vi "DeviceReadStatus.vi"(8 "error in (no error)":errorcluster, 11 "DeviceLoopData in":T1) -> (0 "error out":errorcluster, 1 "Data":variant, 2 "Status":string, 3 "DeviceLoopData out":T1, 4 "Up To Date":bool, 6 "Ready":bool)   [LabVIEW 2015]
uses:
  <vilib>/ErrorRing/Error Ring.xnode
  <vilib>/Utility/error.llb/Error Cluster From Error Code.vi
  NetworkStream/NetworkStreamData.ctl
  DeviceLoopData.ctl
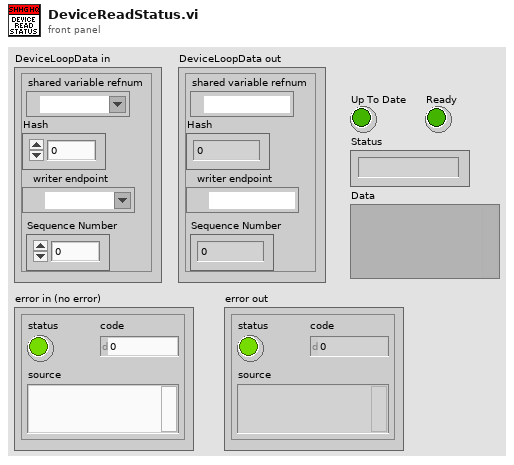
[diagram p1: front panel]
types:
  T1 = typedef "DeviceLoopData.ctl" = cluster{"shared variable refnum":refnum<k21>, "Hash":u64, "writer endpoint":refnum<k21>, "Sequence Number":u64}
  T2 = typedef "NetworkStream.lvlib/NetworkStreamData.ctl" = cluster{"Command/Status":string, "Data":variant, "Session Hash":u64, "Sequence Number":u64}
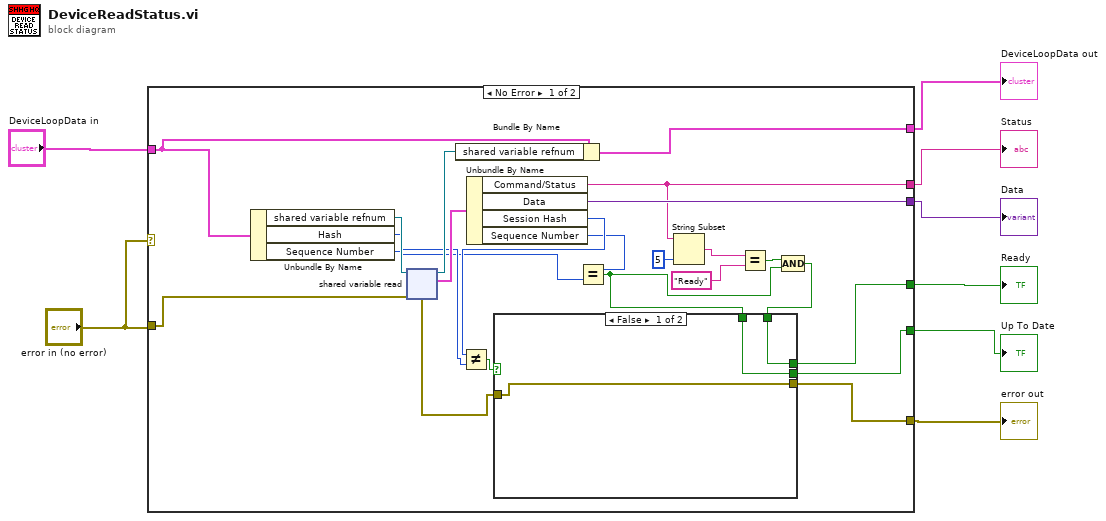
[diagram p0: block diagram]
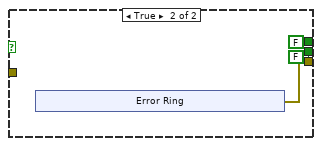
[diagram p2: hidden frame]
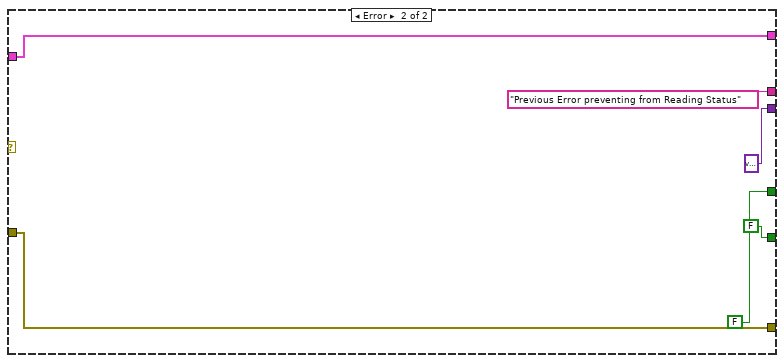
[diagram p3: hidden frame]
diagram:
  n1 = case shown="No Error" "error in (no error)" {
    tunnel: [w23 w48] -> w8
    tunnel: "error in (no error)" -> [w30 w48]
    tunnel: [w20 w46] -> w6
    tunnel: [w13 "Previous Error preventing from Reading Status" ("Command/Status")] -> w5
    tunnel: [w19 variant ("Data")] -> w4
    tunnel: [w10 FALSE] -> w3
    tunnel: "DeviceLoopData in" -> [w18 w46]
    tunnel: [w11 FALSE] -> w1
    frame No Error {
      n2 = Unbundle By Name(w18) -> ("shared variable refnum"=w28:refnum<k21>, "Hash"=w25:u64, "Sequence Number"=w21:u64)
      n3 = shared-variable-read(w28, w30) -> (w31:refnum<k21>, w24:errorcluster, w29:T2)
      n4 = Bundle By Name(cluster=w18, "shared variable refnum"=w31) -> (w20:T1)
      n5 = Unbundle By Name(w29) -> ("Command/Status"=w13:string, "Data"=w19:variant, "Session Hash"=w26:u64, "Sequence Number"=w22:u64)
      n6 = Not Equal?(x=w26, y=w25) -> (x != y?=w27:bool)
      n7 = Equal?(x=w22, y=w21) -> (x = y?=w9:bool)
      n8 = String Subset(string=w13, length (rest)=5 ("length (rest)")) -> (substring=w16:string)  [unwired: 1 in]
      n9 = Equal?(x=w16, y="Ready") -> (x = y?=w14:bool)
      n10 = Compound Arithmetic op=AND(w14, w9) -> (w12:bool)
      n11 = case shown="False" w27 {
        tunnel: w24 -> [w34 _]
        tunnel: [w34 w37] -> w23
        tunnel: w12 -> [w33 _]
        tunnel: [w33 FALSE] -> w11
        tunnel: [w32 FALSE] -> w10
        tunnel: w9 -> [w32 _]
        frame False {
        }
        frame True {
          n12 = xnode "Error Ring"() -> ("error out"=w37:errorcluster)
        }
      }
    }
    frame Error {
    }
  }
  "error out" <- w8
  "Up To Date" <- w3
  "Data" <- w4
  "Status" <- w5
  "DeviceLoopData out" <- w6
  "Ready" <- w1
